vi "Process.vi"(8 "error in (no error)":errorcluster, 10 "Pound in":refnum<class "Pound.lvclass">, 11 "Qbus in":refnum<class "Qbus.lvclass">) -> (0 "error out":errorcluster)   [LabVIEW 2017, in "USBDrive.lvlib"]
uses:
  <vilib>/addons/InsightCM/Devices/Shared/Common/USBDrive/USBDrive.lvlib
  <vilib>/addons/Qbus/Qbus.lvclass
  <vilib>/NI/Software Watchdog/Pound/Pound.lvclass
  <vilib>/addons/InsightCM/Devices/Shared/Common/USBDrive/controls/config.ctl
  <vilib>/addons/TimerProcess/controls/taskType.ctl
  <vilib>/addons/TraceLogger/TraceLogger.lvlib
  <vilib>/NI/Software Watchdog/Watchdog/Watchdog.lvclass
  <vilib>/addons/TimerProcess/TimerProcess.lvlib
  <vilib>/addons/InsightCM/Utilities/GlobalConfiguration/GlobalConfiguration.lvlib
  <vilib>/addons/InsightCM/Utilities/PropertyHelpers/PropertyHelpers.lvlib
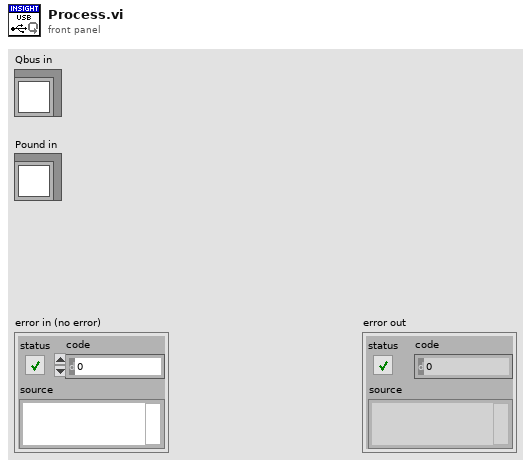
[diagram p1: front panel]
types:
  T1 = typedef "USBDrive.lvlib/config.ctl" = cluster{"USBdrive":path, "USBpresentState":bool}
  T2 = typedef "TimerProcess.lvlib/taskType.ctl" = enum16{"single", "repeat"}
  T3 = typedef "SectionKeyValues.ctl" = cluster{"Section":string, "KeyValues":T4[]}
  T4 = typedef "KeyValuePair.ctl" = cluster{"Key":string, "Value":string}
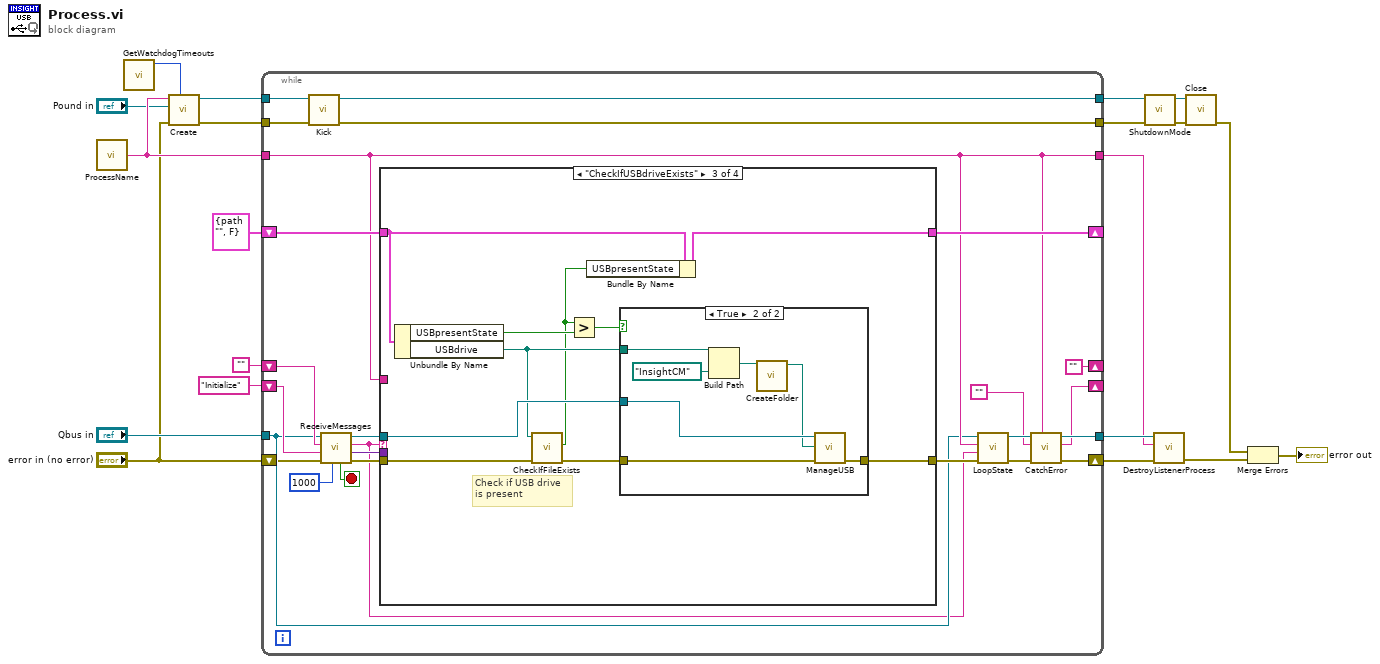
[diagram p0: block diagram]
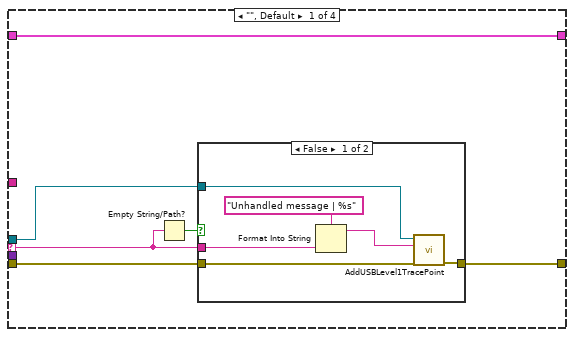
[diagram p2: hidden frame]
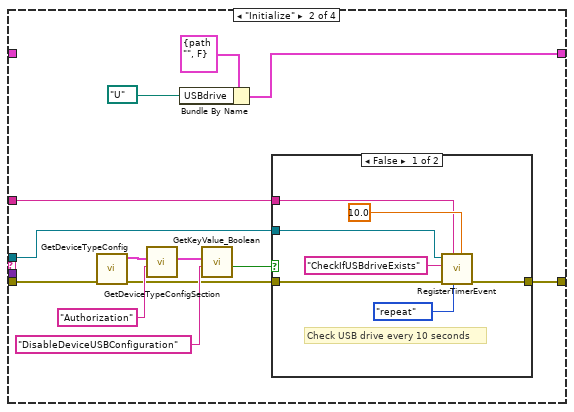
[diagram p4: hidden frame]
diagram:
  n1 = call <vilib>:"ProcessName.vi"() -> ("ProcessName"=w14:string)  [unwired: 5 in]
  n2 = call <vilib>:"GetWatchdogTimeouts.vi"() -> ("software timeout"=w1:u32)  [unwired: 10 in, 1 out]
  n3 = call <vilib>:"Create.vi"("Execution Timeout (ms)"=w1, "error in (no error)"="error in (no error)", "Pound"="Pound in", "Name"=w14) -> ("error out"=w8:errorcluster, "Watchdog"=w13:refnum<data-value>)  [unwired: 6 in]
  n4 = while {
    shift-right: [""] -> _
    shift-left: "" -> [w44]
    tunnel: "Qbus in" -> [w31]
    tunnel: w14 -> [w32]
    tunnel: [w35] -> w18
    tunnel: [w32] -> w17
    shift-right: [w34] -> _
    shift-left: "Initialize" -> [w39]
    shift-right: [w37] -> _
    shift-left: T1 {"USBdrive"=path "", "USBpresentState"=FALSE} ("config") -> [w38]
    tunnel: w13 -> [w30]
    tunnel: [w29] -> w10
    tunnel: w8 -> [w28]
    tunnel: [w26] -> w7
    shift-right: [w36] -> w19
    shift-left: "error in (no error)" -> [w27]
    stop <- w45 stop-if-true
    n5 = call <vilib>:"Kick.vi"("error in (no error)"=w28, "Watchdog"=w30) -> ("error out"=w26:errorcluster, "Watchdog"=w29:refnum<data-value>)  [unwired: 8 in]
    n6 = call <vilib>:"ReceiveMessages.vi"("timeout (1000)"=1000 ("milliseconds to wait"), "error in (no error)"=w27, "priority action"=w39, "default action"=w44, "Qbus in"=w31) -> ("error out"=w43:errorcluster, "message value"=w40:variant, "action"=w25:string, "Qbus out"=w41:refnum<class "Qbus.lvclass">, "exit"=w45:bool)  [unwired: 2 in]
    n7 = case shown="\"CheckIfUSBdriveExists\"" w25 {
      selector: w25 -> [w49 _ _ _]
      tunnel: w43 -> [w48 w63 w89 w98]
      tunnel: w41 -> [w46 w69 w87 _]
      tunnel: [w47 w60 w88 w98] -> w33
      tunnel: w40 -> [_ _ _ _]
      tunnel: w38 -> [w51 _ w83 w99]
      tunnel: [w51 w71 w80 w99] -> w37
      tunnel: w32 -> [_ w68 _ _]
      frame "", Default {
        n8 = Empty String/Path?(string/path=w49) -> (empty?=w50:bool)
        n9 = case shown="False" w50 {
          tunnel: [w54 w58] -> w47
          tunnel: w48 -> [w55 w58]
          tunnel: w49 -> [w57 _]
          tunnel: w46 -> [w53 _]
          frame False {
            n10 = Format Into String(format string="Unhandled message | %s", w57) -> (resulting string=w52:string)  [unwired: 2 in, 1 out]
            n11 = call <vilib>:"AddUSBLevel1TracePoint.vi"("error in (no error)"=w55, "trace log"=w52, "Qbus in"=w53) -> ("error out"=w54:errorcluster)  [unwired: 8 in]
          }
          frame True {
          }
        }
      }
      frame "Initialize" {
        n12 = call <vilib>:"GetDeviceTypeConfig.vi"("error in (no error)"=w63) -> ("error out"=w62:errorcluster, "key values"=w67:T3[])  [unwired: 8 in, 1 out]
        n13 = call <vilib>:"GetDeviceTypeConfigSection.vi"("key"="Authorization", "key values"=w67) -> ("key value pairs out"=w65:T4[])  [unwired: 8 in, 1 out]
        n14 = Bundle By Name(cluster=T1 {"USBdrive"=path "", "USBpresentState"=FALSE} ("config"), "USBdrive"=path "U:/" ("path")) -> (w71:T1)
        n15 = call <vilib>:"GetKeyValue_Boolean.vi"("key"="DisableDeviceUSBConfiguration", "key value pairs"=w65) -> ("value"=w61:bool)  [unwired: 7 in, 2 out]
        n16 = case shown="False" w61 {
          tunnel: w69 -> [w77 _]
          tunnel: w68 -> [w74 _]
          tunnel: w62 -> [w73 w79]
          tunnel: [w72 w79] -> w60
          frame False {
            # "Check USB drive every 10 seconds"
            n17 = call <vilib>:"RegisterTimerEvent.vi"("interval (sec)"=10.0, "type"=taskType."repeat", "process name"=w74, "error in (no error)"=w73, "callback action"="CheckIfUSBdriveExists", "qbus in"=w77) -> ("error out"=w72:errorcluster)  [unwired: 4 in, 1 out]
          }
          frame True {
          }
        }
      }
      frame "CheckIfUSBdriveExists" {
        # "Check if USB drive\nis present"
        n18 = Unbundle By Name(w83) -> ("USBpresentState"=w86:bool, "USBdrive"=w82:path)
        n19 = call <vilib>:"CheckIfFileExists.vi"("error in (no error)"=w89, "path"=w82) -> ("error out"=w85:errorcluster, "file\\folder exists?"=w81:bool)  [unwired: 7 in, 1 out]
        n20 = Greater?(x=w81, y=w86) -> (0:w84:bool)
        n21 = Bundle By Name(cluster=w83, "USBpresentState"=w81) -> (w80:T1)
        n22 = case shown="True" w84 {
          tunnel: w85 -> [w90 w97]
          tunnel: [w90 w96] -> w88
          tunnel: w87 -> [_ w95]
          tunnel: w82 -> [_ w94]
          frame False {
          }
          frame True {
            n23 = Build Path(base path=w94, name or relative path=path "InsightCM" ("path")) -> (appended path=w92:path)
            n24 = call <vilib>:"CreateFolder.vi"("folder"=w92) -> ("folder out"=w91:path)  [unwired: 9 in, 1 out]
            n25 = call <vilib>:"ManageUSB.vi"("error in (no error)"=w97, "USB root"=w91, "Qbus in"=w95) -> ("error out"=w96:errorcluster)  [unwired: 8 in]
          }
        }
      }
      frame "Exit" {
      }
    }
    n26 = call <vilib>:"LoopState.vi"("error in (no error)"=w33, "loop action"=w25, "process name"=w32, "Qbus in"=w31) -> ("error out"=w23:errorcluster, "Qbus out"=w22:refnum<class "Qbus.lvclass">)  [unwired: 6 in]
    n27 = call <vilib>:"CatchError.vi"("source"=w32, "error in (no error)"=w23, "next action in"="", "Qbus in"=w22) -> ("error out"=w36:errorcluster, "next action out"=w34:string, "Qbus out"=w35:refnum<class "Qbus.lvclass">)  [unwired: 5 in]
  }
  n28 = call <vilib>:"ShutdownMode.vi"("error in (no error)"=w7, "Watchdog"=w10) -> ("error out"=w9:errorcluster, "Watchdog"=w11:refnum<data-value>)  [unwired: 8 in]
  n29 = call <vilib>:"DestroyListenerProcess.vi"("error in (no error)"=w19, "process name"=w17, "Qbus in"=w18) -> ("error in (no error)"=w6:errorcluster)  [unwired: 7 in, 1 out]
  n30 = call <vilib>:"Close.vi"("error in (no error)"=w9, "Watchdog"=w11) -> ("error out"=w5:errorcluster)  [unwired: 9 in]
  n31 = Merge Errors(w5, w6) -> (→"error out":errorcluster)
